vi "startMission.vi"(8 "error in (no error)":errorcluster, 11 "StationKeeping in":refnum<class "StationKeeping.lvclass">) -> (0 "error out":errorcluster, 3 "StationKeeping out":refnum<class "StationKeeping.lvclass">)   [LabVIEW 2011, in "StationKeeping.lvclass"]
uses:
  StationKeeping.lvclass
  StationKeeping.lvclass/StationKeeping.ctl
  GenericMission/GenericMission.lvclass
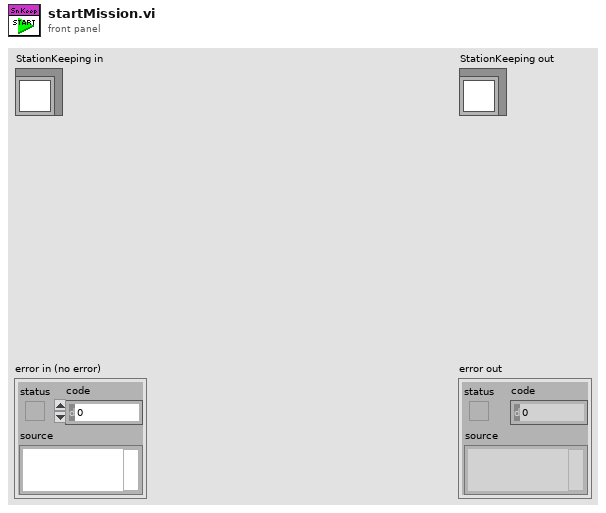
[diagram p1: front panel]
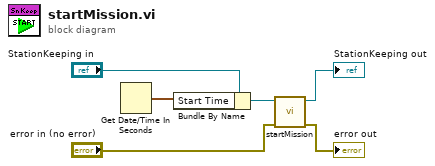
[diagram p0: block diagram]
diagram:
  n1 = Get Date/Time In Seconds() -> (seconds since 1Jan1904=w5:timestamp)
  n2 = Bundle By Name(cluster="StationKeeping in", "Start Time"=w5) -> (w4:refnum<class "StationKeeping.lvclass">)
  n3 = call-parent "startMission.vi"("error in (no error)"="error in (no error)", "GenericMission in"=w4) -> ("error out"=→"error out":errorcluster, "GenericMission out"=→"StationKeeping out":refnum<class "StationKeeping.lvclass">)  [unwired: 8 in]
